vi "Fire Event.vi"(7 "Event Name":string, 8 "error in (no error)":errorcluster, 9 "Event Error":errorcluster, 10 "Event Data":variant, 11 "User Event In":refnum<user-event>) -> (0 "error out":errorcluster, 3 "User Event Out":refnum<user-event>)   [LabVIEW 2011]
doc: "This VI will fire a user event using the <b>Event Name</b>, with <b>Event Data</b>, and <b>Event Error</b>, on the <b>User Event In</b>. It does this by putting all the data for the event into a Variant Repository and firing the event with a Variant data type."
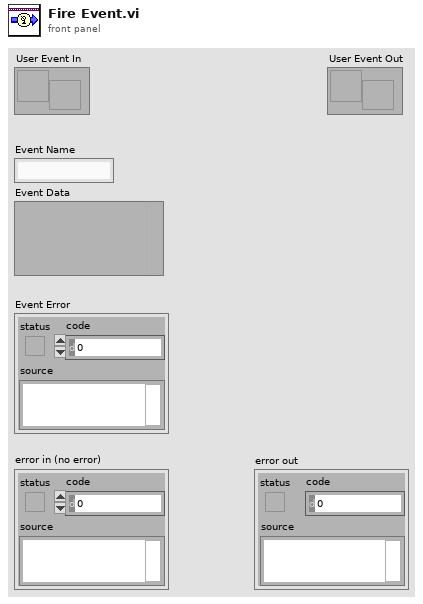
[diagram p1: front panel]
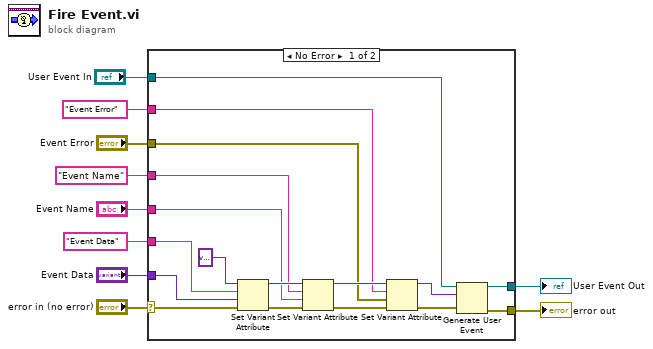
[diagram p0: block diagram]
diagram:
  n1 = case shown="No Error" "error in (no error)" {
    selector: "error in (no error)" -> [w24 w29]
    tunnel: "Event Data" ("Tag") -> [w22 _]
    tunnel: "Event Error" ("Tag") -> [w16 _]
    tunnel: "Event Name" ("Tag") -> [w19 _]
    tunnel: [w27 w28] -> w7
    tunnel: "User Event In" -> [w26 w28]
    tunnel: [w25 w29] -> w5
    tunnel: "Event Data" -> [w23 _]
    tunnel: "Event Name" -> [w18 _]
    tunnel: "Event Error" -> [w15 _]
    frame No Error {
      n2 = Set Variant Attribute(Variant=variant ("variant"), name=w22, value=w23, error in=w24) -> (Variant out=w21:variant, error out=w20:errorcluster)  [unwired: 1 out]
      n3 = Set Variant Attribute(Variant=w21, name=w19, value=w18, error in=w20) -> (Variant out=w17:variant, error out=w14:errorcluster)  [unwired: 1 out]
      n4 = Set Variant Attribute(Variant=w17, name=w16, value=w15, error in=w14) -> (Variant out=w13:variant, error out=w12:errorcluster)  [unwired: 1 out]
      n5 = Generate User Event(user event=w26, event data cluster=w13, error in=w12) -> (user event out=w27:refnum<user-event>, error out=w25:errorcluster)
    }
    frame Error {
    }
  }
  "User Event Out" <- w7
  "error out" <- w5
